vi "TI sbRIO Main (FPGA) pre 4x ADC.vi"() -> ()   [LabVIEW 2013]
uses:
  <vilib>/eio/EIONode/EIONode.xnode
  <vilib>/rvi/eio/common/nirviEmuTemplateMethod_errors.vi
  <vilib>/rvi/FXPMathLib/FxpMul/XNode/nifxpmath_Multiplier.xnode
  <vilib>/rvi/FXPMathLib/sim/FxpSim.dll
  <vilib>/Platform/TimedLoop/XDataNode/wakeup.ctl
  <vilib>/Platform/TimedLoop/XDataNode/XDNodeRunTimeDep.lvlib
  <vilib>/Platform/TimedLoop/XDataNode/nitl_modes.ctl
  <vilib>/Platform/TimedLoop/XDataNode/timing_clust.ctl
  <vilib>/Platform/TimedLoop/XDataNode/XDataNode.xnode
  <vilib>/rvi/FXPMathLib/basic elements/FxpIntAccumulator/subVIs/nifxpmath_IntAccumulator_SimConfig.ctl
  <vilib>/rvi/FXPMathLib/basic elements/FxpIntAccumulator/simVIs/DllFxpIntAccumulator_sub.vi
  <vilib>/rvi/FXPMathLib/basic elements/FxpIntAccumulator/XNode/nifxpmath_IntAccumulator.xnode
  <vilib>/fxp/LVFixedPointOverflowPolicyTypeDef.ctl
  <vilib>/rvi/FXPMathLib/FxpSqrt/subVIs/nifxpmath_Sqrt_SimConfig.ctl
  <vilib>/rvi/FXPMathLib/FxpSqrt/simVIs/DllSqrtTemp_sub.vi
  <vilib>/rvi/FXPMathLib/FxpSqrt/XNode/nifxpmath_Sqrt.xnode
  <vilib>/rvi/Analysis/common/codeGenErrors/XNode/niFpgaXNodeCodeGenErrorHandle.vi
  <vilib>/rvi/Analysis/measure/dc-rms/XNode/niFpgaDC-RMS.xnode
  <vilib>/rvi/Analysis/measure/period/templates/niFPGA Period Edge Direction.ctl
  <vilib>/rvi/Analysis/utilities/niFPGA Threshold Crossing Logic.vi
  <vilib>/rvi/Analysis/measure/period/XNode/niFpgaAnalogPeriod.xnode
  <vilib>/rvi/FXPMathLib/FxpDiv/XNode/nifxpmath_Div.xnode
  <vilib>/rvi/DataTransferAndStorage/Container/XNode/niFpgaContainer.xnode
  <vilib>/rvi/FXPMathLib/FxpAdd/XNode/nifxpmath_Add.xnode
  <vilib>/rvi/FXPMathLib/FxpDiv/simVIs/DllFxpDivTemp_sub.vi
  <vilib>/rvi/FXPMathLib/FxpDiv/subVIs/nifxpmath_Div_SimConfig.ctl
  <vilib>/rvi/interface/RandomDataEmulation/nirviRandomDataFpgaReadWriteTemplate.vi
  <vilib>/rvi/Analysis/measure/butterworth/XNode/niFpgaButterworthFilter.xnode
  Controls/SPI Channels.ctl
  <vilib>/eio/EIOMethodNode/EIOMethodNode.xnode
  <userlib>/_NI SPI IP/FPGA/Controllers/Public/Spi Master Inputs.ctl
  <userlib>/_NI SPI IP/FPGA/Controllers/DIO SPI FPGA.lvlib
  <userlib>/_NI SPI IP/FPGA/Controllers/Public/Transfer Settings.ctl
panel:
  out "AI16-47":fxp<+/-,28,17>[](array[numeric])
  out "ADC Read Data":u64 format="%.0x"
  in  "ADC CS Mode":enum16{"All", "CS0", "CS1"}(ring)
  in  "ADC Trigger":bool=TRUE
  in  "ADC SPI Settings":T1 {"Direction Change Bit" max=64 step=1; "Transfer Length (bits)" min=1 max=64 step=1}
  in  "ADC Data In":u64 format="%.0x"
  in  "ADC Conversion Request":bool
  in  "ADC Manual":bool
  in  "RPMhyst":fxp<+,25,6>=0.39999961853027344
  in  "CommFactor":fxp<+,32,16>
  in  "Brushless":bool
  in  "DIO47":bool
  in  "DIO48":bool
  in  "Reset Starts":bool
  out "Detected Starts":u32[](array[numeric])
  out "AI6-31":fxp<+/-,28,17>[](array[numeric])
  in  "DIO63":bool
  out "AI24-31":fxp<+/-,28,17>[](array[numeric])
  out "AI16-23":fxp<+/-,28,17>[](array[numeric])
  in  "AI Divisor":u32
  in  "AO3":fxp<+/-,20,5>
  in  "AO2":fxp<+/-,20,5>
  in  "AO1":fxp<+/-,20,5>
  in  "AO0":fxp<+/-,20,5>
  out "Actual Loop Time":u32
  in  "Loop Timer (uSec)":u32=100
  out "Elapsed Times":fxp<+,40,40>[](array[numeric]) format="%.30g"
  in  "Timer Resets":bool[](array[boolean])=[FALSE, FALSE, FALSE, FALSE, FALSE, FALSE]
  out "Speed (RPM)":fxp<+/-,28,17>[](array[numeric])
  out "Pump Currents":fxp<+/-,28,17>[](array[numeric])
  in  "Duty (Ticks) 6":i32
  in  "Duty (Ticks) 5":i32
  in  "Duty (Ticks) 4":i32
  in  "Duty (Ticks) 3":i32
  in  "PWM Period (Ticks)":u32=40000000
  in  "Duty (Ticks) 1":i32
  in  "Duty (Ticks) 2":i32
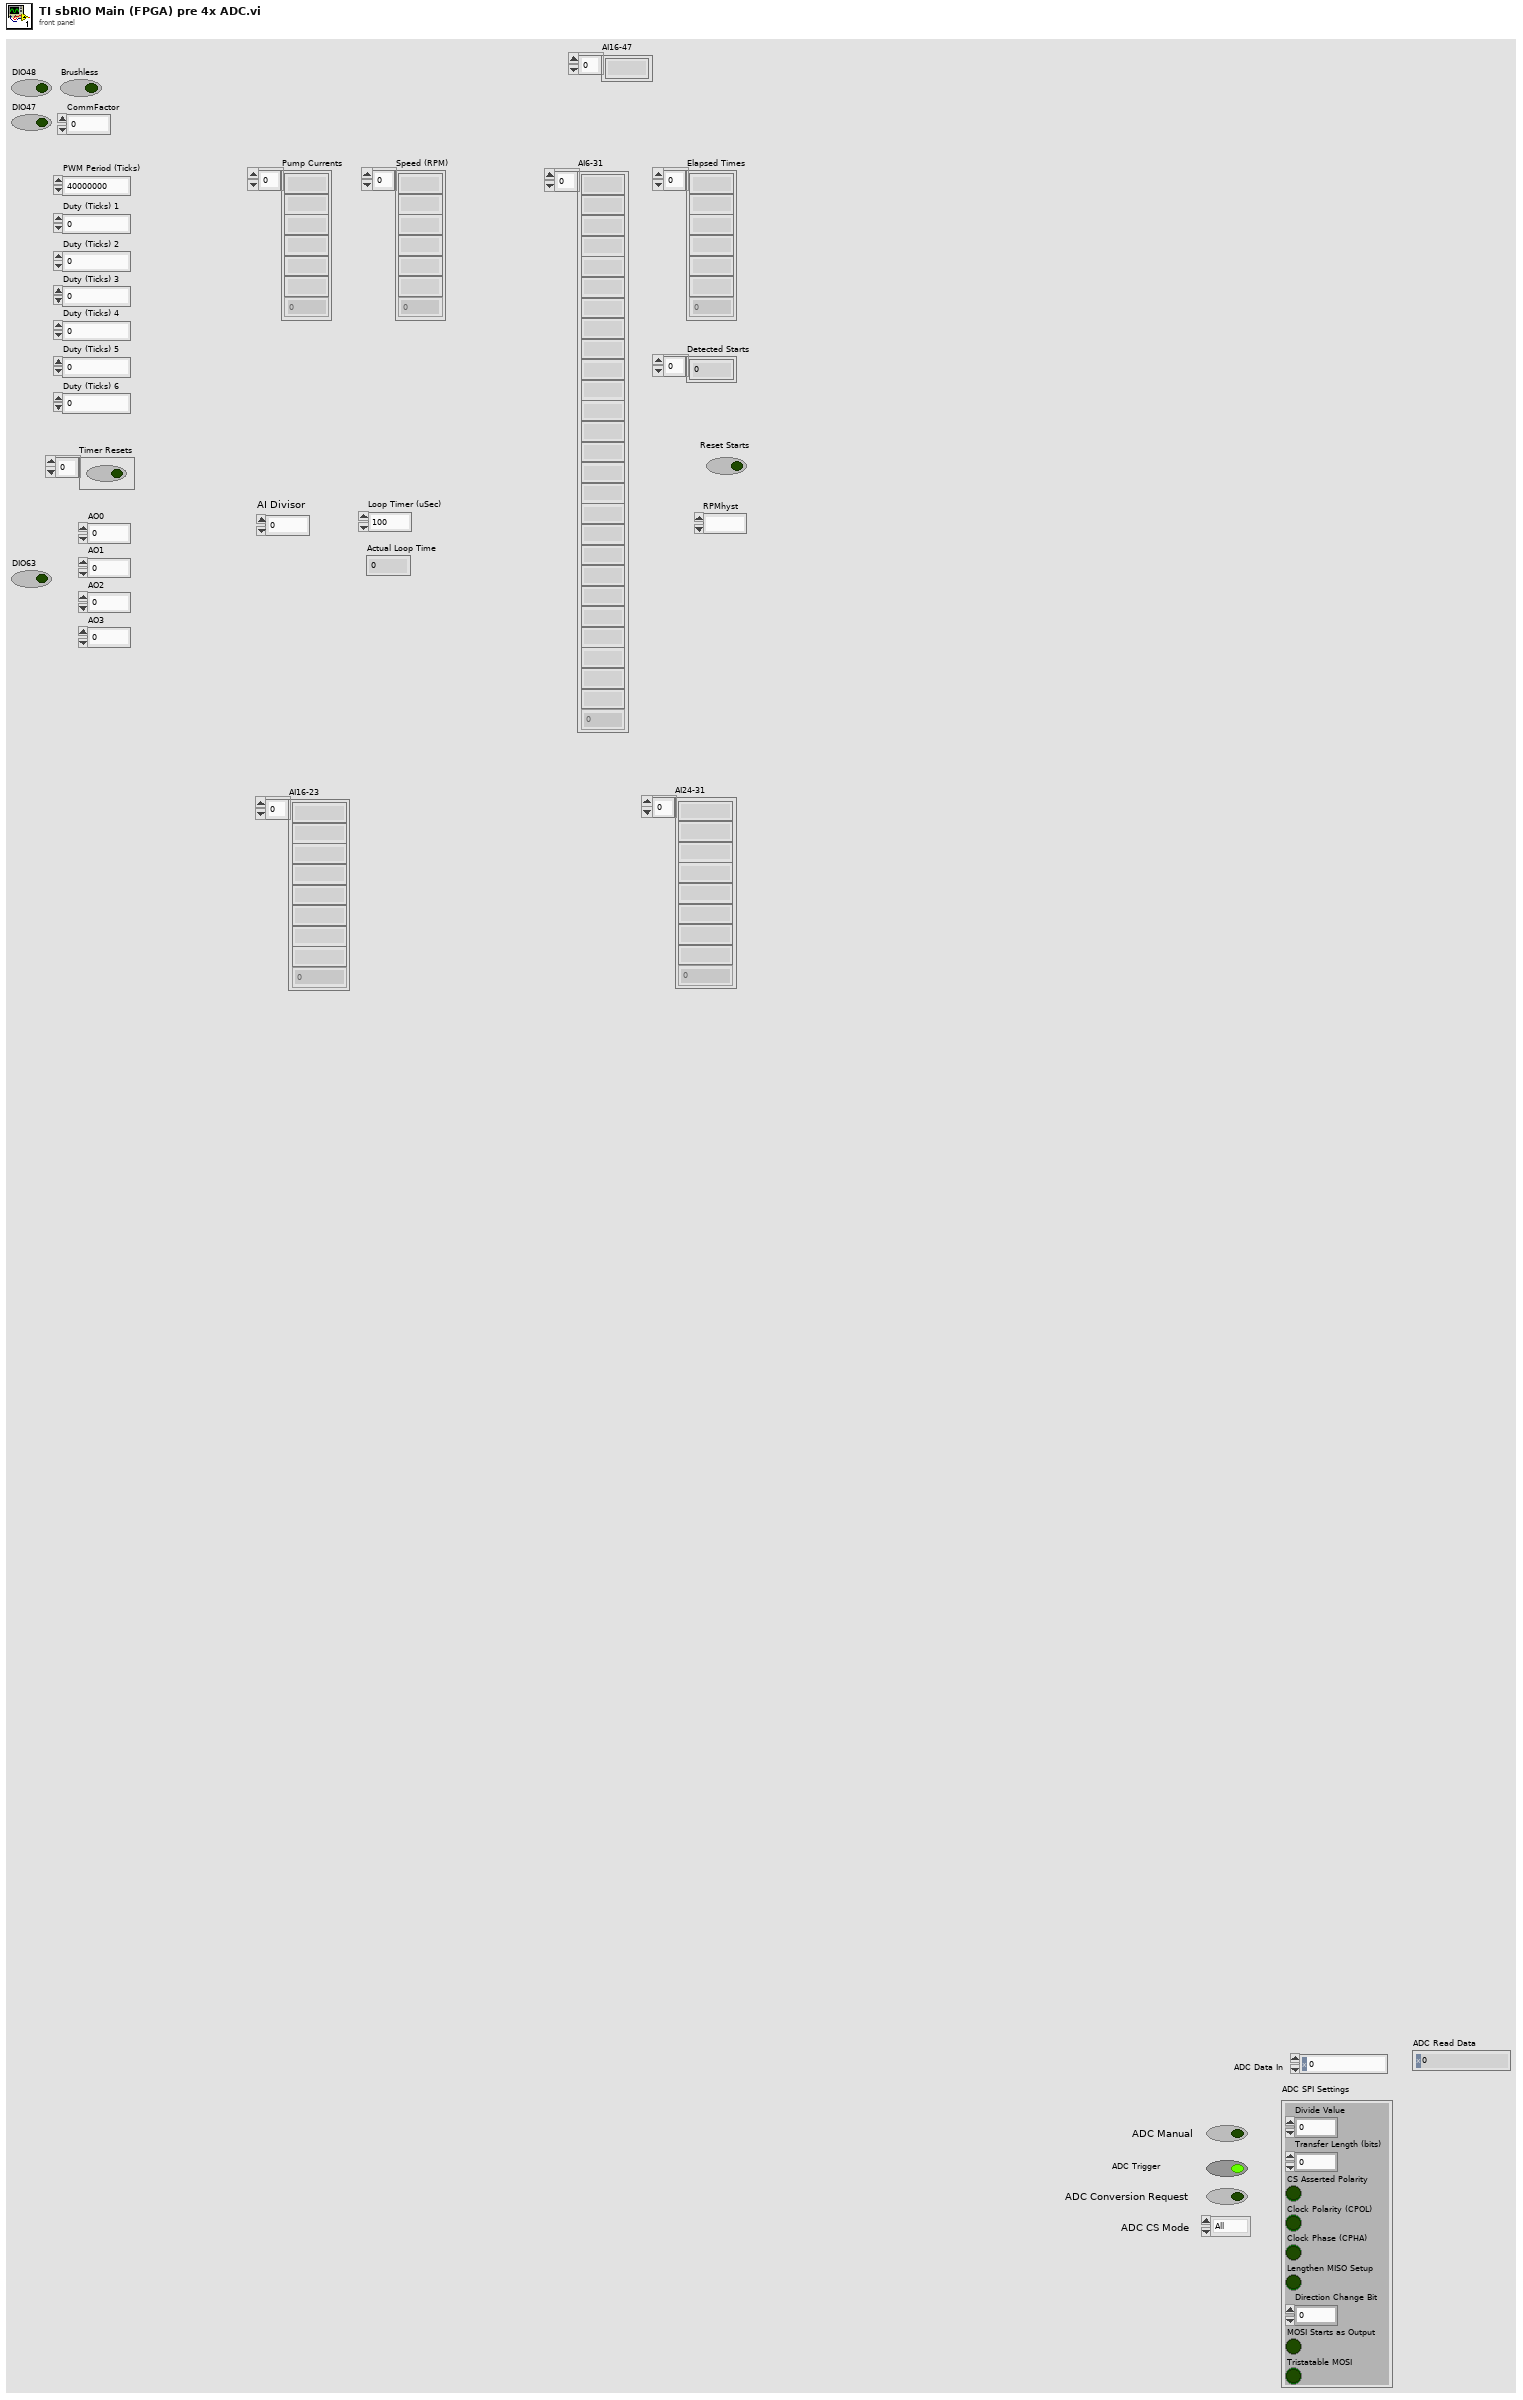
[diagram p1: front panel]
types:
  T1 = typedef "DIO SPI FPGA.lvlib/Transfer Settings.ctl" = cluster{"Divide Value":u8, "Transfer Length (bits)":u8, "CS Asserted Polarity":bool, "Clock Polarity (CPOL)":bool, "Clock Phase (CPHA)":bool, "Lengthen MISO Setup":bool, "Direction Change Bit":u8, "MOSI Starts as Output":bool, "Tristatable MOSI":bool}
  T2 = typedef "SPI Channels.ctl" = cluster{"CS":refnum<k21>, "CLK":refnum<k21>, "MOSI":refnum<k21>, "MISO":refnum<k21>}
  T3 = typedef "XDNodeRunTimeDep.lvlib/timing_clust.ctl" = cluster{"Expected End [f-1]":u64, "Actual End [f-1]":u64, "Finished Late? [f-1]":bool, "Expected End [i-1]":u64, "Actual End [i-1]":u64, "Finished Late? [i-1]":bool, "Expected Start [i]":u64, "Actual Start [i]":u64, "Expected Start [f]":u64, "Actual Start [f]":u64, "Source Name":string, "Structure Name":string, "Period":i64, "Deadline":i64, "Offset":i64, "Start":i64, "Priority":i32, "Timeout":i32, "Mode":T4, "Wakeup Reason":T5, "Error":errorcluster, "Source Type":string, "Secondary Source Type":string, "Global End Time":u64, "Global Start Time":u64, "Frame Duration":u64, "Iteration Duration":u64, "Assigned CPU":i32, "I/O Scan Engine Mode":u32}
  T4 = typedef "XDNodeRunTimeDep.lvlib/nitl_modes.ctl" = enum32{"No Change", "Process missed periods, maintain original phase", "Discard missed periods, maintain original phase", "Process missed periods, ignore original phase", "Discard missed periods, ignore original phase"}
  T5 = typedef "XDNodeRunTimeDep.lvlib/wakeup.ctl" = enum32{"Normal", "Aborted", "Asynchronous wakeup", "Timing source error", "Timed loop error", "Timeout"}
  T6 = typedef "DIO SPI FPGA.lvlib/Spi Master Inputs.ctl" = cluster{"MISO":bool}
  T7 = typedef "DIO SPI FPGA.lvlib/Spi Master Outputs.ctl" = cluster{"Chip Select":bool, "Clock":bool, "MOSI":bool, "MOSI OE":bool}
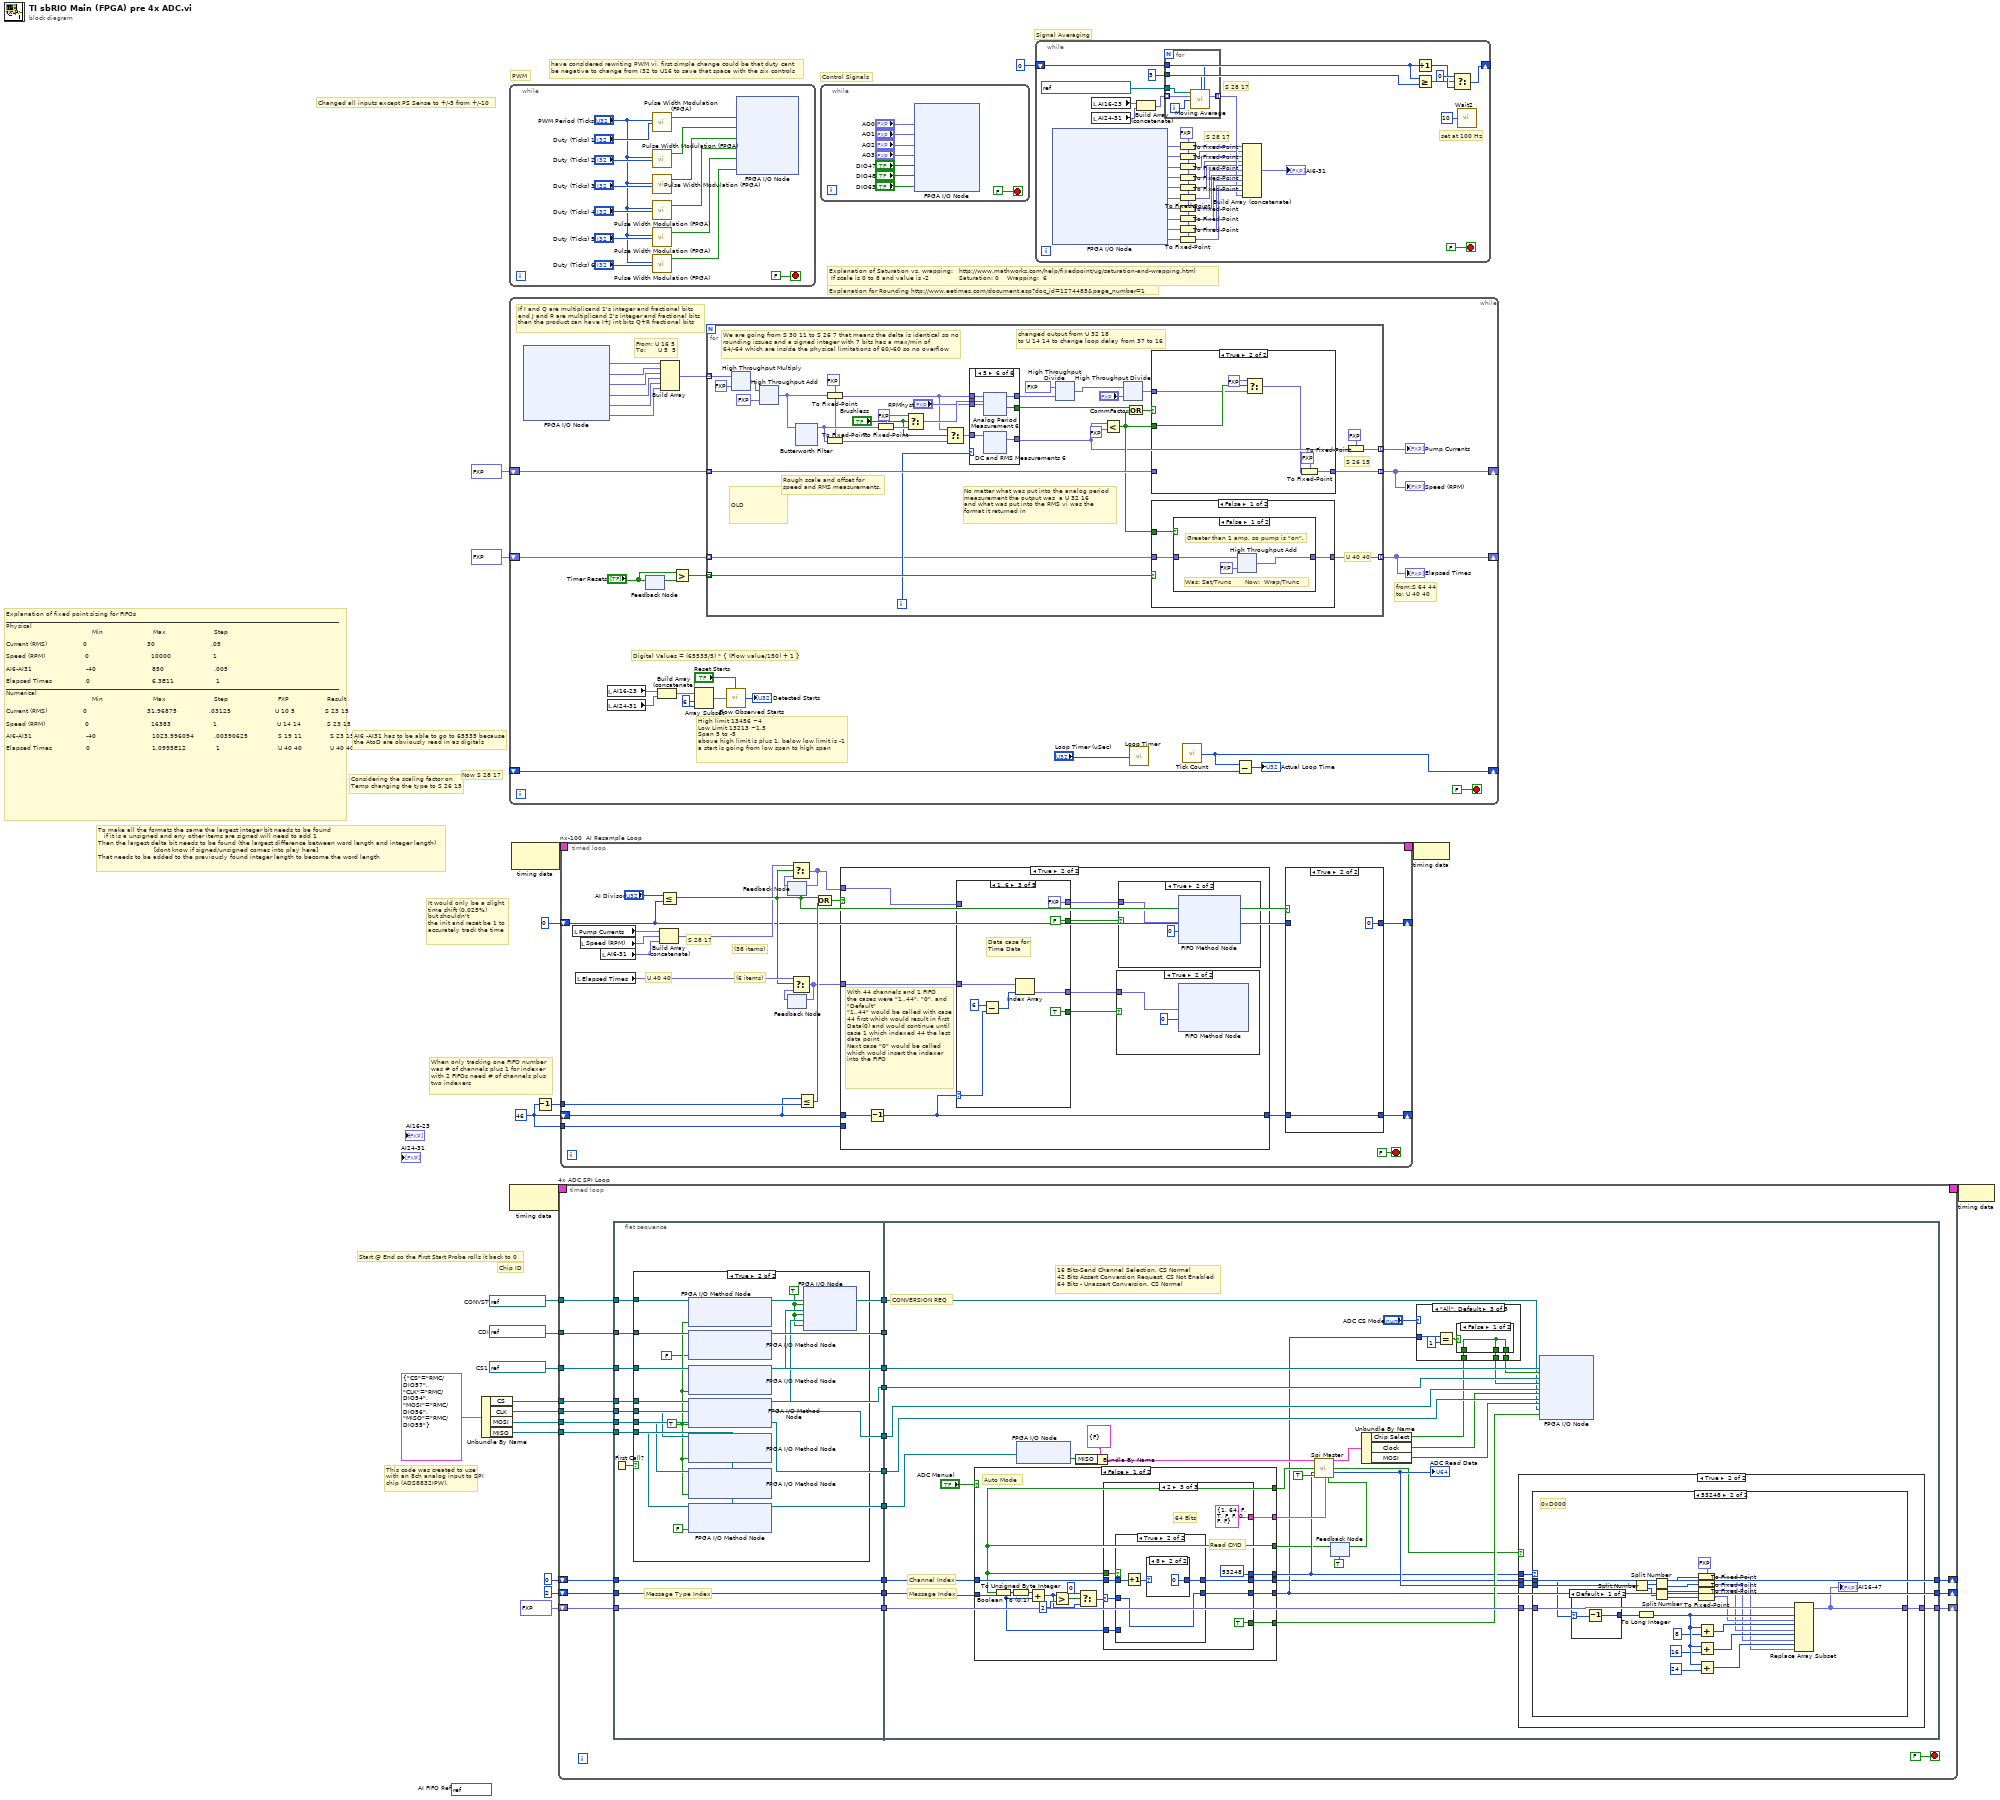
[diagram p0: block diagram]
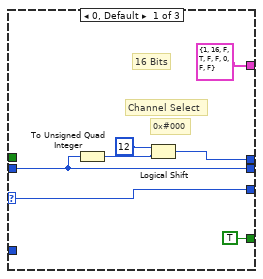
[diagram p3: hidden frame]
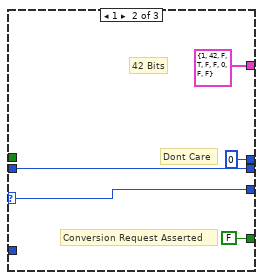
[diagram p4: hidden frame]
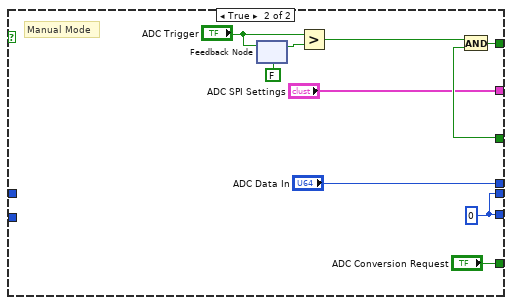
[diagram p7: hidden frame]
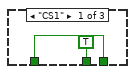
[diagram p8: hidden frame]
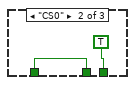
[diagram p9: hidden frame]
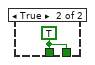
[diagram p10: hidden frame]
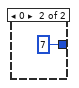
[diagram p13: hidden frame]
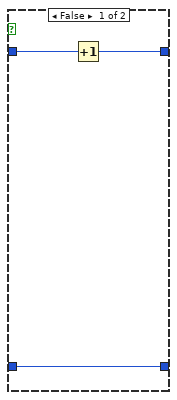
[diagram p14: hidden frame]
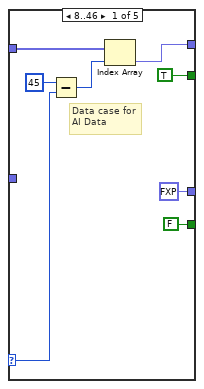
[diagram p18: hidden frame]
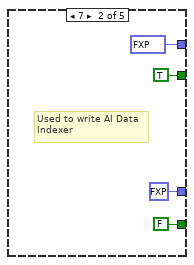
[diagram p19: hidden frame]
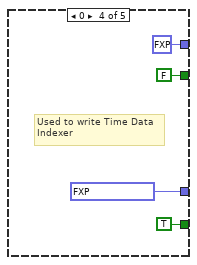
[diagram p20: hidden frame]
diagram:
  w9 = refnum<k21> "RMC/DIO60"  # CONVST
  w10 = refnum<k21> "RMC/DIO59"  # CDI
  w11 = refnum<k21> "RMC/DIO58"  # CS1
  (unwired) refnum<k21> "AI Data"  # AI FIFO Ref
  w16 = u32 46 ("Sample Divisor")
  # "Start @ End so the First Start Probe rolls it back to 0"
  # "Chip ID"
  # "This code was created to use\nwith an 8ch analog input to SPI\nchip (ADS8832IPW)."
  # "have considered rewriting PWM vi, first simple change could be that duty cant\nbe negative to change from I32 to U16 to save that space with the six controls"
  # "PWM"
  # "Changed all inputs except PS Sense to +/-5 from +/-10"
  # "Explanation for Rounding http://www.eetimes.com/document.asp?doc_id=1274485&page_number=1"
  # "Explanation of Saturation vs. wrapping:   http://www.mathworks.com/help/fixedpoint/ug/saturation-and-wrapping.html\n If scale is 0 to 8 and value is -2               Saturation: 0    Wrapping:  6"
  # "Control Signals"
  # "Now S 28 17"
  # "AI6 -AI31 has to be able to go to 65535 because\nthe AtoD are obviously read in as digitals"
  # "When only tracking one FIFO number\nwas # of channels plus 1 for indexer\nwith 2 FIFOs need # of channels plus\ntwo indexers"
  # "It would only be a slight\ntime shift (0.025%)\nbut shouldn't\nthe init and reset be 1 to\naccurately track the time"
  # "Considering the scaling factor on\nTemp changing the type to S 26 15"
  # "Explanation of fixed point sizing for FIFOs\n_______________________________________________________________________________________________________________\nPhysical\n                                           Min                         Max                        Step\n\nCurrent (RMS)                  0                              30                            .05                      \n\nSpeed (RPM)                    0                               10000                     1\n\nAI6-AI31                           -40                            850                         .005\n\nElapsed Times                 0                               6.3E11                     1\n_______________________________________________________________________________________________________________\nNumerical\n                                           Min                         Max                        Step                         FXP                   Result\n\nCurrent (RMS)                  0                              31.96875                .03125                      U 10 5               S 23 15\n\nSpeed (RPM)                    0                               16383                     1                              U 14 14             S 23 15\n\nAI6-AI31                           -40                            1023.996094          .00390625               S 19 11              S 23 15\n\nElapsed Times                 0                               1.0995E12               1                             U 40 40              U 40 40"
  # "To make all the formats the same the largest integer bit needs to be found\n   if it is a unsigned and any other items are signed will need to add 1\nThen the largest delta bit needs to be found (the largest difference between word length and integer length)\n                            [dont know if signed/unsigned comes into play here]\nThat needs to be added to the previously found integer length to become the word length"
  # "Signal Averaging"
  n1 = Unbundle By Name(T2 {"CS"="RMC/DIO57", "CLK"="RMC/DIO54", "MOSI"="RMC/DIO56", "MISO"="RMC/DIO55"} ("SPI Channels")) -> ("CS"=w2:refnum<k21>, "CLK"=w3:refnum<k21>, "MOSI"=w4:refnum<k21>, "MISO"=w5:refnum<k21>)
  n2 = while {
    stop <- FALSE stop-if-true
    n3 = call "Pulse Width Modulation (FPGA).vi"("PWM Period (Ticks)"="PWM Period (Ticks)", "PWM Duty Cycle (Ticks)"="Duty (Ticks) 1") -> ("PWM DO"=w34:bool)  [unwired: 14 in, 3 out]
    n4 = call "Pulse Width Modulation (FPGA).vi"("PWM Period (Ticks)"="PWM Period (Ticks)", "PWM Duty Cycle (Ticks)"="Duty (Ticks) 2") -> ("PWM DO"=w31:bool)  [unwired: 14 in, 3 out]
    n5 = call "Pulse Width Modulation (FPGA).vi"("PWM Period (Ticks)"="PWM Period (Ticks)", "PWM Duty Cycle (Ticks)"="Duty (Ticks) 3") -> ("PWM DO"=w25:bool)  [unwired: 14 in, 3 out]
    n6 = call "Pulse Width Modulation (FPGA).vi"("PWM Period (Ticks)"="PWM Period (Ticks)", "PWM Duty Cycle (Ticks)"="Duty (Ticks) 4") -> ("PWM DO"=w24:bool)  [unwired: 14 in, 3 out]
    n7 = call "Pulse Width Modulation (FPGA).vi"("PWM Period (Ticks)"="PWM Period (Ticks)", "PWM Duty Cycle (Ticks)"="Duty (Ticks) 5") -> ("PWM DO"=w23:bool)  [unwired: 14 in, 3 out]
    n8 = call "Pulse Width Modulation (FPGA).vi"("PWM Period (Ticks)"="PWM Period (Ticks)", "PWM Duty Cycle (Ticks)"="Duty (Ticks) 6") -> ("PWM DO"=w22:bool)  [unwired: 14 in, 3 out]
    n9 = xnode "FPGA I/O Node"("RMC/DIO0"=w34, "RMC/DIO1"=w31, "RMC/DIO2"=w25, "RMC/DIO3"=w24, "RMC/DIO4"=w23, "RMC/DIO5"=w22) -> ()  [unwired: 7 in, 7 out]
  }
  n10 = while {
    shift-right: [w46] -> _
    shift-left: fxp<+,28,17>[] [0.0, 0.0, 0.0, 0.0, 0.0, 0.0] -> [w48]
    shift-right: [w47] -> _
    shift-left: fxp<+,40,40>[] [0.0, 0.0, 0.0, 0.0, 0.0, 0.0] -> [w50]
    shift-right: [w53] -> _
    shift-left: _ -> [w52]
    stop <- FALSE stop-if-true
    w41 = 6 ("index")
    # "High limit 13456 ~4\nLow Limit 13213 ~1.5\nSpan 5 to -5\nabove high limit is plus 1, below low limit is -1\na start is going from low span to high span"
    # "Digital Values = (65535/5) * { (Flow value/150) + 1 }"
    # "from:S 64 44\nto: U 40 40"
    # "From: U 16 5\nTo:      U 5  5"
    # "If I and Q are multiplicand 1's integer and fractional bits\nand J and R are multiplicand 2's integer and fractional bits\nthen the product can have I+J int bits Q+R fractional bits"
    n11 = xnode "FPGA I/O Node"() -> ("Voltage_1 (AI0/8)"=w56:fxp<+/-,24,5>, "Voltage_2 (AI1/9)"=w62:fxp<+/-,24,5>, "Voltage_3 (AI2/10)"=w61:fxp<+/-,24,5>, "Voltage_4 (AI3/11)"=w60:fxp<+/-,24,5>, "Voltage_5 (AI4/12)"=w59:fxp<+/-,24,5>, "Voltage_6 (AI5/13)"=w58:fxp<+/-,24,5>)  [unwired: 6 in, 6 out]
    n12 = local read "AI16-23"() -> (w43:fxp<+/-,28,17>[])
    n13 = local read "AI24-31"() -> (w44:fxp<+/-,28,17>[])
    n14 = feedback #1() -> (w36:bool[])  [unwired: 1 in]
    n15 = feedback-in #1("Timer Resets") -> ()
    n16 = Build Array (concatenate)(w43, w44) -> (w42:fxp<+/-,28,17>[])
    n17 = Build Array(w56, w62, w61, w60, w59, w58) -> (w45:fxp<+/-,24,5>[])
    n18 = Greater?(x="Timer Resets", y=w36) -> (0:w54:bool[])
    n19 = Array Subset(array=w42, index=w41, length=w41) -> (w40:fxp<+/-,28,17>[])
    n20 = for {
      tunnel: w45 -> [w87] mode=indexing
      tunnel: w48 -> [w92] mode=indexing
      tunnel: [w79] -> w46 mode=indexing
      tunnel: w54 -> [w90] mode=indexing
      tunnel: [w80] -> w49 mode=indexing
      tunnel: w50 -> [w84] mode=indexing
      tunnel: [w83] -> w47 mode=indexing
      i -> [w89]
      w77 = fxp<+/-,24,7> 0.0 ("threshold level")
      w63 = fxp<+/-,26,7> 0.0 ("out")
      # "OLD"
      # "U 40 40"
      # "S 26 15"
      # "changed output from U 32 18\nto U 14 14 to change loop delay from 37 to 16"
      # "No matter what was put into the analog period\nmeasurement the output was  a U 32 16\nand what was put into the RMS vi was the\nformat it returned in"
      # "We are going from S 30 11 to S 26 7 that means the delta is identical so no\nrounding issues and a signed integer with 7 bits has a max/min of\n64/-64 which are inside the physical limitations of 60/-60 so no overflow"
      # "Rough scale and offset for\nspeed and RMS measurements."
      n21 = xnode ("High Throughput Multiply")("x"=w87, "y"=fxp<+,5,5> 24.0 ("Current Scale")) -> ("x*y"=w88:fxp<+/-,29,10>)
      n22 = xnode ("High Throughput Add")("x"=w88, "y"=fxp<+/-,7,7> -60.0 ("Current Offset")) -> ("x+y"=w78:fxp<+/-,30,11>)
      n23 = xnode "Butterworth Filter"("input data"=w78) -> ("output data"=w65:fxp<+/-,20,15>)  [unwired: 2 in, 1 out]
      n24 = To Fixed-Point(fixed-point type=w63, number=w78) -> (fixed-point=w67:fxp<+/-,26,7>)
      n25 = To Fixed-Point(fixed-point type=w63, number=w65) -> (fixed-point=w64:fxp<+/-,26,7>)
      n26 = To Fixed-Point(fixed-point type=w77, number=w65) -> (fixed-point=w70:fxp<+/-,24,7>)
      n27 = Select(t=w77, s="Brushless", f=w70) -> (s? t:f=w72:fxp<+/-,24,7>)
      n28 = Select(t=w67, s="Brushless", f=w64) -> (s? t:f=w68:fxp<+/-,26,7>)
      n29 = case shown="5" w89 {
        tunnel: [w180 w410 w640 w870 w1100 w1330] -> w82
        tunnel: [w179 w409 w639 w869 w1099 w1329] -> w73
        tunnel: [w178 w408 w638 w868 w1098 w1328] -> w71
        tunnel: w67 -> [w177 w407 w637 w867 w1097 w1327]
        tunnel: w72 -> [w176 w406 w636 w866 w1096 w1326]
        tunnel: "RPMhyst" -> [w175 w405 w635 w865 w1095 w1325]
        tunnel: w68 -> [w174 w404 w634 w864 w1094 w1324]
        frame 0, Default {
          n30 = xnode ("Analog Period Measurement 5")("input data"=w177, "threshold level"=w176, "hysteresis"=w175) -> ("period (samples)"=w178:fxp<+,32,16>, "output valid"=w179:bool)  [unwired: 2 in, 2 out]
          n31 = xnode ("DC and RMS Measurements 5")("input data"=w174) -> ("RMS"=w180:fxp<+,26,7>)  [unwired: 1 in, 1 out]
        }
        frame 1 {
          n32 = xnode ("Analog Period Measurement")("input data"=w407, "threshold level"=w406, "hysteresis"=w405) -> ("period (samples)"=w408:fxp<+,32,16>, "output valid"=w409:bool)  [unwired: 2 in, 2 out]
          n33 = xnode ("DC and RMS Measurements")("input data"=w404) -> ("RMS"=w410:fxp<+,26,7>)  [unwired: 1 in, 1 out]
        }
        frame 2 {
          n34 = xnode ("Analog Period Measurement 2")("input data"=w637, "threshold level"=w636, "hysteresis"=w635) -> ("period (samples)"=w638:fxp<+,32,16>, "output valid"=w639:bool)  [unwired: 2 in, 2 out]
          n35 = xnode ("DC and RMS Measurements 2")("input data"=w634) -> ("RMS"=w640:fxp<+,26,7>)  [unwired: 1 in, 1 out]
        }
        frame 3 {
          n36 = xnode ("Analog Period Measurement 3")("input data"=w867, "threshold level"=w866, "hysteresis"=w865) -> ("period (samples)"=w868:fxp<+,32,16>, "output valid"=w869:bool)  [unwired: 2 in, 2 out]
          n37 = xnode ("DC and RMS Measurements 3")("input data"=w864) -> ("RMS"=w870:fxp<+,26,7>)  [unwired: 1 in, 1 out]
        }
        frame 4 {
          n38 = xnode ("Analog Period Measurement 4")("input data"=w1097, "threshold level"=w1096, "hysteresis"=w1095) -> ("period (samples)"=w1098:fxp<+,32,16>, "output valid"=w1099:bool)  [unwired: 2 in, 2 out]
          n39 = xnode ("DC and RMS Measurements 4")("input data"=w1094) -> ("RMS"=w1100:fxp<+,26,7>)  [unwired: 1 in, 1 out]
        }
        frame 5 {
          n40 = xnode ("Analog Period Measurement 6")("input data"=w1327, "threshold level"=w1326, "hysteresis"=w1325) -> ("period (samples)"=w1328:fxp<+,32,16>, "output valid"=w1329:bool)  [unwired: 2 in, 2 out]
          n41 = xnode ("DC and RMS Measurements 6")("input data"=w1324) -> ("RMS"=w1330:fxp<+,26,7>)  [unwired: 1 in, 1 out]
        }
      }
      n42 = xnode "High Throughput Divide"("x"=fxp<+,14,19> 300000.0, "y"=w71) -> ("x/y"=w76:fxp<+,18,16>)
      n43 = Less?(x=w82, y=fxp<+,26,7> 1.0 ("current threshold")) -> (x < y?=w91:bool)
      n44 = xnode "High Throughput Divide"("x"=w76, "y"="CommFactor") -> ("x/y"=w74:fxp<+,14,14>)
      n45 = Or(x=w73, y=w91) -> (x .or. y?=w93:bool)
      n46 = case shown="True" w93 {
        tunnel: w74 -> [_ w144]
        tunnel: w91 -> [_ w145]
        tunnel: w92 -> [w140 _]
        tunnel: [w140 w141] -> w79
        frame False {
        }
        frame True {
          n47 = Select(t=fxp<+,14,14> 0.0 ("input data"), s=w145, f=w144) -> (s? t:f=w142:fxp<+,14,14>)
          n48 = To Fixed-Point(fixed-point type=fxp<+/-,28,17> 0.0 ("out"), number=w142) -> (fixed-point=w141:fxp<+/-,28,17>)
        }
      }
      n49 = case shown="False" w90 {
        tunnel: w91 -> [w98 _]
        tunnel: w84 -> [w97 _]
        tunnel: [w96 fxp<+,40,40> 0.0 ("AI0")] -> w83
        frame False {
          n50 = case shown="False" w98 {
            tunnel: [w99 w102] -> w96
            tunnel: w97 -> [w101 w102]
            frame False {
              # "Was: Sat/Trunc       Now:  Wrap/Trunc"
              # "Greater than 1 amp, so pump is \"on\"."
              n51 = xnode ("High Throughput Add")("x"=w101, "y"=fxp<+,1,1> 1.0) -> ("x+y"=w99:fxp<+,40,40>)
            }
            frame True {
            }
          }
        }
        frame True {
        }
      }
      n52 = To Fixed-Point(fixed-point type=fxp<+/-,28,17> 0.0 ("out"), number=w82) -> (fixed-point=w80:fxp<+/-,28,17>)
    }
    "Pump Currents" <- w49
    "Speed (RPM)" <- w46
    "Elapsed Times" <- w47
    n53 = call "Flow Observed Starts.vi"("Reset Starts"="Reset Starts", "Flows"=w40) -> ("Observed Starts"=→"Detected Starts":u32[])  [unwired: 13 in]
    n54 = call "Loop Timer"("Count(uSec)"="Loop Timer (uSec)") -> ()  [unwired: 1 out]
    n55 = call "Tick Count"() -> ("Tick Count(uSec)"=w53:u32)
    n56 = Subtract(x=w53, y=w52) -> (x-y=→"Actual Loop Time":u32)
  }
  n57 = node-c288() -> (w13:T3)  [unwired: 1 in]
  n58 = node-c288() -> (w20:T3)  [unwired: 1 in]
  n59 = Decrement(x=w16) -> (x-1=w17:u32)
  n60 = timed-loop "4x ADC SPI Loop" {
    shift-right: [w1575] -> _
    shift-left: fxp<+/-,28,17>[] [0.0, 0.0, 0.0, 0.0, 0.0, 0.0, 0.0, 0.0, 0.0, 0.0, 0.0, 0.0, 0.0, 0.0, 0.0, 0.0, 0.0, 0.0, 0.0, 0.0, 0.0, 0.0, 0.0, 0.0, 0.0, 0.0, 0.0, 0.0, 0.0, 0.0, 0.0, 0.0] -> [w1576]
    tunnel: w2 -> [w1574]
    tunnel: w3 -> [w1573]
    tunnel: w4 -> [w1572]
    tunnel: w5 -> [w1571]
    tunnel: w11 -> [w1570]
    tunnel: w9 -> [w1569]
    tunnel: w10 -> [w1568]
    timing: w13 -> [_]
    timing-out: [_] -> w12
    shift-right: [w1557] -> _
    shift-left: u8 2 ("lo(x)") -> [w1558]
    shift-right: [w1554] -> _
    shift-left: u8 0 ("lo(x)") -> [w1555]
    stop <- FALSE stop-if-true
    n61 = flat-sequence {
      tunnel: [w1587] -> w1567
      tunnel: w1576 -> [w1587]
      tunnel: w1574 -> [w1586]
      tunnel: w1573 -> [w1585]
      tunnel: w1572 -> [w1584]
      tunnel: w1571 -> [w1583]
      tunnel: [w1586] -> w1566
      tunnel: [w1585] -> w1565
      tunnel: [w1584] -> w1564
      tunnel: [w1583] -> w1563
      tunnel: w1570 -> [w1582]
      tunnel: w1569 -> [w1581]
      tunnel: w1568 -> [w1580]
      tunnel: [w1582] -> w1562
      tunnel: [w1580] -> w1561
      tunnel: [w1581] -> w1560
      tunnel: [w1579] -> w1559
      tunnel: w1558 -> [w1579]
      tunnel: [w1578] -> w1556
      tunnel: w1555 -> [w1578]
      tunnel: w1567 -> [w1630]
      tunnel: [w1629] -> w1575
      tunnel: w1566 -> [w1625]
      tunnel: w1565 -> [w1628]
      tunnel: w1564 -> [w1627]
      tunnel: w1563 -> [w1626]
      tunnel: w1562 -> [w1624]
      tunnel: w1561 -> [_]
      tunnel: w1560 -> [w1610]
      tunnel: w1559 -> [w1611]
      tunnel: [w1605] -> w1557
      tunnel: w1556 -> [w1604]
      tunnel: [w1603] -> w1554
      frame #0 {
        # "Message Type Index"
        n62 = First Call?() -> (First Call?: T/F=w1588:bool)
        n63 = case shown="True" w1588 {
          tunnel: w1586 -> [_ w1601]
          tunnel: w1585 -> [_ w1600]
          tunnel: w1584 -> [_ w1599]
          tunnel: w1583 -> [_ w1598]
          tunnel: w1582 -> [_ w1597]
          tunnel: w1581 -> [_ w1596]
          tunnel: w1580 -> [_ w1594]
          frame False {
          }
          frame True {
            w1589 = TRUE ("I/O Item")
            w1595 = TRUE ("Enable")
            n64 = xnode "FPGA I/O Method Node"("FPGA I/O In"=w1596, "Enable"=w1595) -> ("FPGA I/O Out"=w1590:refnum<k21>)
            n65 = xnode "FPGA I/O Method Node"("FPGA I/O In"=w1594, "Enable"=FALSE) -> ()  [unwired: 1 out]
            n66 = xnode "FPGA I/O Method Node"("FPGA I/O In"=w1597, "Enable"=w1595) -> ("FPGA I/O Out"=w1593:refnum<k21>)
            n67 = xnode "FPGA I/O Method Node"("FPGA I/O In"=w1601, "Enable"=w1595) -> ("FPGA I/O Out"=w1592:refnum<k21>)
            n68 = xnode "FPGA I/O Method Node"("FPGA I/O In"=w1600, "Enable"=w1595) -> ()  [unwired: 1 out]
            n69 = xnode "FPGA I/O Method Node"("FPGA I/O In"=w1599, "Enable"=w1595) -> ()  [unwired: 1 out]
            n70 = xnode "FPGA I/O Method Node"("FPGA I/O In"=w1598, "Enable"=FALSE) -> ()  [unwired: 1 out]
            n71 = xnode "FPGA I/O Node"("I/O Item"=w1589, "FPGA I/O In"=w1590, "I/O Item"=w1589, "FPGA I/O In"=w1593, "I/O Item"=w1589, "FPGA I/O In"=w1592) -> ()  [unwired: 3 out]
          }
        }
      }
      frame #1 {
        # "Message Index"
        # "Channel Index"
        # "16 Bits-Send Channel Selection, CS Normal \n42 Bits Assert Conversion Request, CS Not Enabled\n64 Bits - Unassert Conversion, CS Normal"
        # "CONVERSION REQ"
        n72 = xnode "FPGA I/O Node"("FPGA I/O In"=w1626) -> ("I/O Item"=w1631:bool)  [unwired: 1 out]
        n73 = Bundle By Name(cluster=T6 {"MISO"=FALSE} ("spi input"), "MISO"=w1631) -> (w1632:T6)
        n74 = feedback #2(TRUE ("Chip Select")) -> (w1607:bool)
        n75 = case shown="False" "ADC Manual" {
          tunnel: w1607 -> [w1638 w1685]
          tunnel: [w1638 w1684] -> w1613
          tunnel: [w1643 "ADC SPI Settings"] -> w1612
          tunnel: w1611 -> [w1637 _]
          tunnel: [w1639 "ADC Data In"] -> w1608
          tunnel: [w1636 w1680] -> w1605
          tunnel: [w1642 "ADC Conversion Request"] -> w1609
          tunnel: w1604 -> [w1641 _]
          tunnel: [w1640 w1680] -> w1603
          frame False {
            # "Auto Mode"
            n76 = Boolean To (0,1)(Boolean=w1638) -> (0, 1=w1650:i16)
            n77 = To Unsigned Byte Integer(number=w1650) -> (unsigned 8bit integer=w1649:u8)
            n78 = Add(x=w1649, y=w1637) -> (x+y=w1645:u8)
            n79 = Greater?(x=w1645, y=u8 2) -> (0:w1647:bool)
            n80 = Select(t=u8 0 ("y"), s=w1647, f=w1645) -> (s? t:f=w1644:u8)
            n81 = case shown="2" w1644 {
              selector: w1644 -> [w1654 w1658 w1666]
              tunnel: [T1 {"Divide Value"=1, "Transfer Length (bits)"=16, "CS Asserted Polarity"=FALSE, "Clock Polarity (CPOL)"=TRUE, "Clock Phase (CPHA)"=FALSE, "Lengthen MISO Setup"=FALSE, "Direction Change Bit"=0, "MOSI Starts as Output"=FALSE, "Tristatable MOSI"=FALSE} ("Master Settings 2") T1 {"Divide Value"=1, "Transfer Length (bits)"=42, "CS Asserted Polarity"=FALSE, "Clock Polarity (CPOL)"=TRUE, "Clock Phase (CPHA)"=FALSE, "Lengthen MISO Setup"=FALSE, "Direction Change Bit"=0, "MOSI Starts as Output"=FALSE, "Tristatable MOSI"=FALSE} ("Master Settings 2") T1 {"Divide Value"=1, "Transfer Length (bits)"=64, "CS Asserted Polarity"=FALSE, "Clock Polarity (CPOL)"=TRUE, "Clock Phase (CPHA)"=FALSE, "Lengthen MISO Setup"=FALSE, "Direction Change Bit"=0, "MOSI Starts as Output"=FALSE, "Tristatable MOSI"=FALSE} ("Master Settings 2")] -> w1643
              tunnel: [TRUE ("I/O Item") FALSE ("I/O Item") TRUE ("I/O Item")] -> w1642
              tunnel: w1641 -> [w1653 w1659 w1665]
              tunnel: [w1653 w1659 w1664] -> w1640
              tunnel: [w1651 u64 0 u64 53248] -> w1639
              tunnel: w1638 -> [_ _ w1668]
              tunnel: w1637 -> [_ _ w1663]
              tunnel: [w1654 w1658 w1667] -> w1636
              frame 0, Default {
                # "16 Bits"
                # "Channel Select"
                # "0x#000"
                n82 = To Unsigned Quad Integer(1:w1653) -> (0:w1652:u64)
                n83 = Logical Shift(y=i16 12, x=w1652) -> (x << y=w1651:u64)
              }
              frame 1 {
                # "Conversion Request Asserted"
                # "42 Bits"
                # "Dont Care"
              }
              frame 2 {
                # "64 Bits"
                # "Read CMD"
                n84 = case shown="True" w1668 {
                  tunnel: [w1672 w1676] -> w1667
                  tunnel: w1666 -> [_ w1676]
                  tunnel: w1665 -> [w1673 w1677]
                  tunnel: [w1673 w1674] -> w1664
                  tunnel: w1663 -> [w1672 _]
                  frame False {
                  }
                  frame True {
                    n85 = Increment(x=w1677) -> (x+1=w1675:u8)
                    n86 = case shown="8" w1675 {
                      selector: w1675 -> [w1678 _]
                      tunnel: [w1678 u8 0] -> w1674
                      frame Default {
                      }
                      frame 8 {
                      }
                    }
                  }
                }
              }
            }
          }
          frame True {
            w1680 = u8 0 ("y")
            # "Manual Mode"
            n87 = feedback #3(FALSE) -> (w1689:bool)
            n88 = feedback-in #3("ADC Trigger") -> ()
            n89 = Greater?(x="ADC Trigger", y=w1689) -> (0:w1686:bool)
            n90 = And(x=w1686, y=w1685) -> (x .and. y?=w1684:bool)
          }
        }
        n91 = call <userlib>:"Spi Master.vi"("spi input"=w1632, "start strobe"=w1613, "data to write"=w1608, "MOSI output enable done"=TRUE, "spi transfer settings"=w1612) -> ("spi output"=w1635:T7, "read data valid"=w1606:bool, "read data"=w1620:u64, "ready for input"=w1622:bool)  [unwired: 7 in]
        "ADC Read Data" <- w1620
        n92 = feedback-in #2(w1622) -> ()
        n93 = Unbundle By Name(w1635) -> ("Chip Select"=w1617:bool, "Clock"=w1621:bool, "MOSI"=w1634:bool)
        n94 = case shown="\"All\", Default" "ADC CS Mode" {
          tunnel: w1617 -> [w1691 w1693 w1697]
          tunnel: [TRUE ("Chip Select") w1693 w1696] -> w1616
          tunnel: [w1691 TRUE ("Chip Select") w1695] -> w1615
          tunnel: w1605 -> [_ _ w1699]
          frame "CS1" {
          }
          frame "CS0" {
          }
          frame "All", Default {
            n95 = Equal?(x=w1699, y=u8 1) -> (x = y?=w1694:bool)
            n96 = case shown="False" w1694 {
              tunnel: w1697 -> [w1700 _]
              tunnel: [w1700 w1701] -> w1696
              tunnel: [w1700 w1701] -> w1695
              frame False {
              }
              frame True {
                w1701 = TRUE ("Chip Select")
              }
            }
          }
        }
        n97 = case shown="True" w1606 {
          tunnel: w1620 -> [_ w1707]
          tunnel: w1630 -> [w1702 w1706]
          tunnel: [w1702 w1705] -> w1629
          tunnel: w1608 -> [_ w1704]
          tunnel: w1603 -> [_ w1703]
          frame False {
          }
          frame True {
            n98 = case shown="53248" w1704 {
              tunnel: w1707 -> [_ w1731]
              tunnel: w1706 -> [w1708 w1729]
              tunnel: [w1708 w1730] -> w1705
              tunnel: w1703 -> [_ w1718]
              frame Default {
              }
              frame 53248 {
                w1717 = fxp<+/-,28,17> 0.0 ("AI0")
                # "0xD000"
                n99 = case shown="Default" w1718 {
                  selector: w1718 -> [w1732 _]
                  tunnel: [w1733 u8 7] -> w1719
                  frame Default {
                    n100 = Decrement(x=w1732) -> (x-1=w1733:u8)
                  }
                  frame 0 {
                  }
                }
                n101 = Split Number(x=w1731) -> (hi(x)=w1728:u32, lo(x)=w1727:u32)
                n102 = To Long Integer(number=w1719) -> (32bit integer=w1726:i32)
                n103 = Split Number(x=w1728) -> (hi(x)=w1713:u16, lo(x)=w1714:u16)
                n104 = Split Number(x=w1727) -> (hi(x)=w1715:u16, lo(x)=w1716:u16)
                n105 = To Fixed-Point(fixed-point type=w1717, number=w1713) -> (fixed-point=w1709:fxp<+/-,28,17>)
                n106 = To Fixed-Point(fixed-point type=w1717, number=w1714) -> (fixed-point=w1710:fxp<+/-,28,17>)
                n107 = To Fixed-Point(fixed-point type=w1717, number=w1715) -> (fixed-point=w1711:fxp<+/-,28,17>)
                n108 = To Fixed-Point(fixed-point type=w1717, number=w1716) -> (fixed-point=w1712:fxp<+/-,28,17>)
                n109 = Add(x=w1726, y=8) -> (x+y=w1724:i32)
                n110 = Add(x=w1726, y=16) -> (x+y=w1723:i32)
                n111 = Add(x=w1726, y=24) -> (x+y=w1722:i32)
                n112 = Replace Array Subset(array=w1729, new element #1=w1712, index #1=w1726, new element #2=w1711, index #2=w1724, new element #3=w1710, index #3=w1723, new element #4=w1709, index #4=w1722) -> (w1730:fxp<+/-,28,17>[])
                "AI16-47" <- w1730
              }
            }
          }
        }
        n113 = xnode "FPGA I/O Node"("I/O Item"=w1615, "FPGA I/O In"=w1624, "I/O Item"=w1616, "FPGA I/O In"=w1625, "I/O Item"=w1621, "FPGA I/O In"=w1628, "I/O Item"=w1634, "FPGA I/O In"=w1627, "I/O Item"=w1609, "FPGA I/O In"=w1610) -> ()  [unwired: 5 out]
      }
    }
  }
  n114 = timed-loop "nx-100  AI Resample Loop" {
    timing: w20 -> [_]
    timing-out: [_] -> w19
    shift-right: [w1756] -> _
    shift-left: u32 0 ("Sample Divisor") -> [w1738]
    shift-right: [w1755] -> _
    shift-left: w16 -> [w1739]
    tunnel: w17 -> [w1749]
    tunnel: w16 -> [w1748]
    stop <- FALSE stop-if-true
    # "(38 items)"
    # "(6 items)"
    # "S 28 17"
    # "U 40 40"
    n115 = local read "Pump Currents"() -> (w1746:fxp<+/-,28,17>[])
    n116 = local read "Elapsed Times"() -> (w1744:fxp<+,40,40>[])
    n117 = local read "Speed (RPM)"() -> (w1747:fxp<+/-,28,17>[])
    n118 = local read "AI6-31"() -> (w1737:fxp<+/-,28,17>[])
    n119 = Build Array (concatenate)(w1746, w1747, w1737) -> (w1740:fxp<+/-,28,17>[])
    n120 = Less Or Equal?(x="AI Divisor", y=w1738) -> (x <= y?=w1743:bool)
    n121 = feedback #4() -> (w1751:fxp<+/-,28,17>[])  [unwired: 1 in]
    n122 = feedback #5() -> (w1745:fxp<+,40,40>[])  [unwired: 1 in]
    n123 = Select(t=w1740, s=w1743, f=w1751) -> (s? t:f=w1750:fxp<+/-,28,17>[])
    n124 = feedback-in #4(w1750) -> ()
    n125 = Select(t=w1744, s=w1743, f=w1745) -> (s? t:f=w1742:fxp<+,40,40>[])
    n126 = feedback-in #5(w1742) -> ()
    n127 = Less Or Equal?(x=w1739, y=w1749) -> (x <= y?=w1753:bool)
    n128 = Or(x=w1743, y=w1753) -> (x .or. y?=w1741:bool)
    n129 = case shown="True" w1741 {
      tunnel: w1739 -> [_ w1768]
      tunnel: [w1763 w1769] -> w1752
      tunnel: w1750 -> [_ w1764]
      tunnel: w1748 -> [w1763 _]
      tunnel: w1742 -> [_ w1767]
      frame False {
      }
      frame True {
        # "With 44 channels and 1 FIFO\nthe cases were \"1..44\", \"0\", and\n\"Default\"\n\"1..44\" would be called with case\n44 first which would result in first\nData(0) and would continue until\ncase 1 which indexed 44 the last\ndata point\nNext case \"0\" would be called\nwhich would insert the indexer\ninto the FIFO"
        n130 = Decrement(x=w1768) -> (x-1=w1769:u32)
        n131 = case shown="1..6" w1769 {
          selector: w1769 -> [w1780 _ w1788 _ _]
          tunnel: [w1778 fxp<+/-,28,17> -9999.0 ("AI0") fxp<+/-,28,17> 0.0 ("AI0") fxp<+/-,28,17> 0.0 ("AI0") fxp<+/-,28,17> -5000.0 ("AI0")] -> w1771
          tunnel: [TRUE TRUE FALSE FALSE FALSE] -> w1770
          tunnel: w1764 -> [w1782 _ _ _ _]
          tunnel: w1767 -> [_ _ w1791 _ _]
          tunnel: [fxp<+,40,40> 0.0 ("AI0") fxp<+,40,40> 0.0 ("AI0") w1790 fxp<+,40,40> 1099511627775.0 ("AI0") fxp<+,40,40> 1099511627774.0 ("AI0")] -> w1766
          tunnel: [FALSE FALSE TRUE TRUE FALSE] -> w1765
          frame 8..46 {
            # "Data case for\nAI Data"
            n132 = Subtract(x=u32 45 ("Sample Divisor"), y=w1780) -> (x-y=w1779:u32)
            n133 = Index Array(array=w1782, index=w1779) -> (element=w1778:fxp<+/-,28,17>)
          }
          frame 7 {
            # "Used to write AI Data\nIndexer"
          }
          frame 1..6 {
            # "Data case for\nTime Data"
            n134 = Subtract(x=u32 6 ("Sample Divisor"), y=w1788) -> (x-y=w1794:u32)
            n135 = Index Array(array=w1791, index=w1794) -> (element=w1790:fxp<+,40,40>)
          }
          frame 0 {
            # "Used to write Time Data\nIndexer"
          }
          frame Default {
            # "Sould never get to\nthis case."
          }
        }
        n136 = case shown="True" w1765 {
          tunnel: w1766 -> [_ w1773]
          frame False {
          }
          frame True {
            n137 = xnode ("FIFO Method Node")("Element"=w1773, "Timeout"=0) -> ()  [unwired: 1 in, 2 out]
          }
        }
        n138 = case shown="True" w1770 {
          tunnel: w1771 -> [_ w1775]
          frame False {
          }
          frame True {
            n139 = xnode ("FIFO Method Node")("Element"=w1775, "Timeout"=0) -> ()  [unwired: 1 in, 2 out]
          }
        }
      }
    }
    n140 = case shown="True" w1743 {
      tunnel: w1738 -> [w1760 _]
      tunnel: [w1759 u32 0] -> w1756
      tunnel: w1752 -> [w1758 w1761]
      tunnel: [w1758 w1761] -> w1755
      frame False {
        n141 = Increment(x=w1760) -> (x+1=w1759:u32)
      }
      frame True {
      }
    }
  }
  n142 = while {
    stop <- FALSE stop-if-true
    n143 = xnode "FPGA I/O Node"("AO0"="AO0", "AO1"="AO1", "AO2"="AO2", "AO3"="AO3", "RMC/DIO47"="DIO47", "RMC/DIO48"="DIO48", "RMC/DIO63"="DIO63") -> ()  [unwired: 8 in, 8 out]
  }
  n144 = while {
    shift-right: [w1842] -> _
    shift-left: 0 ("Moving Point Index") -> [w1843]
    stop <- FALSE stop-if-true
    w1820 = fxp<+/-,28,17> 0.0 ("Controller_Current_1 (AI6)")
    w1841 = 5 ("N (# of Ave Pts 8 max)")
    # "S 28 17"
    # "S 24 5"
    # "S 28 17"
    # "set at 100 Hz"
    n145 = xnode "FPGA I/O Node"() -> ("Spare_1"=w1826:fxp<+/-,24,5>, "Spare_3"=w1825:fxp<+/-,24,5>, "Controller_Current_3 (AI8)"=w1824, "Controller_Current_4 (AI9)"=w1823, "Controller_Current_5 (AI10)"=w1822, "Controller_Current_6 (AI11)"=w1821, "Spare_1 (AI12)"=w1831, "Temp_1 (AI13)"=w1830, "Spare_2"=w1829:fxp<+/-,24,5>, "PS_Sense (AI15)"=w1828:fxp<+/-,24,5>)  [unwired: 10 in, 10 out]
    n146 = local read "AI16-23"() -> (w1832:fxp<+/-,28,17>[])
    n147 = local read "AI24-31"() -> (w1840:fxp<+/-,28,17>[])
    n148 = Build Array (concatenate)(w1832, w1840) -> (w1839:fxp<+/-,28,17>[])
    n149 = for {
      tunnel: w1843 -> [w1849]
      tunnel: w1841 -> [w1850]
      tunnel: [w1854] -> w1833 mode=indexing
      tunnel: w1839 -> [w1853] mode=indexing
      tunnel: refnum<k21> "Running Avg Memory" ("Memory") -> [w1852]
      i -> [w1851]
      n150 = call "Moving Average.vi"("Memory In"=w1852, "N (# of Ave Pts 8 max)"=w1850, "Moving Point Index"=w1849, "Data IN"=w1853, "Channel#"=w1851) -> ("Averaged Data"=w1854:fxp<+/-,28,17>)  [unwired: 10 in]
    }
    n151 = To Fixed-Point(fixed-point type=w1820, number=w1826) -> (fixed-point=w1814:fxp<+/-,28,17>)
    n152 = To Fixed-Point(fixed-point type=w1820, number=w1825) -> (fixed-point=w1815:fxp<+/-,28,17>)
    n153 = To Fixed-Point(fixed-point type=w1820, number=w1824) -> (fixed-point=w1816:fxp<+/-,28,17>)
    n154 = To Fixed-Point(fixed-point type=w1820, number=w1823) -> (fixed-point=w1817:fxp<+/-,28,17>)
    n155 = To Fixed-Point(fixed-point type=w1820, number=w1822) -> (fixed-point=w1818:fxp<+/-,28,17>)
    n156 = To Fixed-Point(fixed-point type=w1820, number=w1821) -> (fixed-point=w1819:fxp<+/-,28,17>)
    n157 = To Fixed-Point(fixed-point type=w1820, number=w1831) -> (fixed-point=w1838:fxp<+/-,28,17>)
    n158 = To Fixed-Point(fixed-point type=w1820, number=w1830) -> (fixed-point=w1837:fxp<+/-,28,17>)
    n159 = To Fixed-Point(fixed-point type=w1820, number=w1829) -> (fixed-point=w1836:fxp<+/-,28,17>)
    n160 = To Fixed-Point(fixed-point type=w1820, number=w1828) -> (fixed-point=w1835:fxp<+/-,28,17>)
    n161 = Build Array (concatenate)(w1814, w1815, w1816, w1817, w1818, w1819, w1838, w1837, w1836, w1835, w1833) -> (→"AI6-31":fxp<+/-,28,17>[])
    n162 = Increment(x=w1843) -> (x+1=w1845:i32)
    n163 = Greater Or Equal?(x=w1843, y=w1841) -> (x >= y?=w1844:bool)
    n164 = Select(t=0, s=w1844, f=w1845) -> (s? t:f=w1842:i32)
    n165 = call "Wait2"("Count(mSec)"=u32 10) -> ()  [unwired: 1 out]
  }
  n166 = node-c288(w19) -> ()
  n167 = node-c288(w12) -> ()
